vi "readFromXML.vi"(8 "error in (no error)":errorcluster, 10 "XML in":string, 11 "FocusSelect in":refnum<class "FocusSelect.lvclass">) -> (0 "error out":errorcluster, 3 "FocusSelect out":refnum<class "FocusSelect.lvclass">)   [LabVIEW 2014, in "TCSDataDefinitions.lvlib" / "TCSCommand.lvlib" / "FocusSelect.lvclass"]
uses:
  FocusSelect.lvclass
  Enumerations/FocusNameTypes.ctl
  FocusSelect.lvclass/FocusSelect.ctl
  TCSTcsCommand/TCSTcsCommand.lvclass
  TCSCommand.lvlib
panel:
  out "focusName":T1
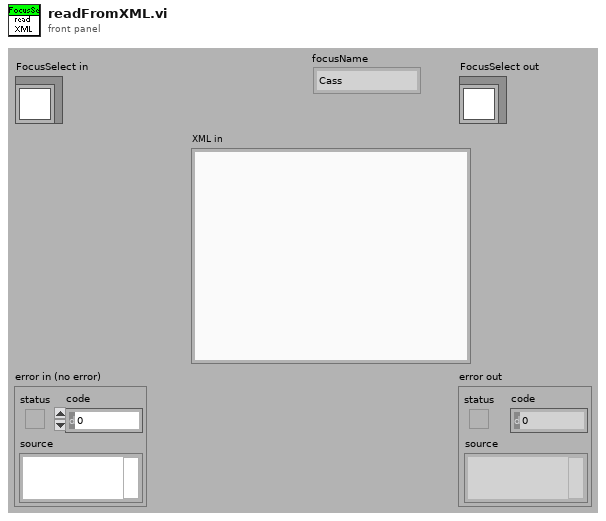
[diagram p1: front panel]
types:
  T1 = typedef "TCSDataDefinitions.lvlib/TCSCommand.lvlib/FocusNameTypes.ctl" = enum16{"Cass", "Prime", "Nasmyth1", "Nasmyth2", "BentCass1", "BentCass2", "BentCass3", "BentCass4", "BentCass5", "BentCass6"}
  T2 = typedef "XML element list.ctl" = T3[]
  T3 = typedef "XML element.ctl" = cluster{"name":string, "contents":string}
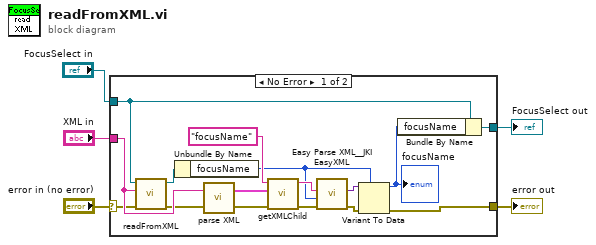
[diagram p0: block diagram]
diagram:
  n1 = case shown="No Error" "error in (no error)" {
    selector: "error in (no error)" -> [w7 w22]
    tunnel: [w11 w23] -> w3
    tunnel: "FocusSelect in" -> [w10 w23]
    tunnel: "XML in" -> [w8 _]
    tunnel: [w12 w22] -> w1
    frame No Error {
      n2 = call-parent "readFromXML.vi"("error in (no error)"=w7, "XMLin"=w8, "TCSTcsCommand in"=w10) -> ("error out"=w6:errorcluster, "TCSTcsCommand out"=w9:refnum<class "FocusSelect.lvclass">)  [unwired: 7 in]
      n3 = Unbundle By Name(w9) -> ("focusName"=w14:T1)
      n4 = call "parse XML.vi"("error in (no error)"=w6, "XMLString in"=w8) -> ("error out"=w21:errorcluster, "XML element list out"=w20:T2)
      n5 = call "getXMLChild.vi"("error in (no error)"=w21, "XML element list in"=w20, "ChildName"="focusName") -> ("error out"=w17:errorcluster, "XML content string out"=w18:string)  [unwired: 6 in, 1 out]
      n6 = call <vilib>:"Easy Parse XML__JKI EasyXML.vi"("error in (no error)"=w17, "LabVIEW Data (Type)"=w14, "XML String"=w18) -> ("error out"=w16:errorcluster, "LabVIEW Data"=w15:variant)  [unwired: 7 in]
      n7 = Variant To Data(error in=w16, type=w14, Variant=w15) -> (data=w13:T1, error out=w12:errorcluster)
      "focusName" <- w13
      n8 = Bundle By Name(cluster=w10, "focusName"=w13) -> (w11:refnum<class "FocusSelect.lvclass">)
    }
    frame Error {
    }
  }
  "error out" <- w1
  "FocusSelect out" <- w3
